vi "unregisterObserverEvent.vi"(8 "error in":errorcluster, 9 "EventReg":refnum<event-registration>, 11 "ObserverClass in":refnum<class "ObserverClass.lvclass">) -> (0 "error out":errorcluster, 3 "ObserverClass out":refnum<class "ObserverClass.lvclass">)   [LabVIEW 2025, in "ObserverClass.lvlib" / "ObserverClass.lvclass"]
doc: "Unregister Observer Event for each Observable"
uses:
  ObserverClass.lvclass
  Controls/observerControl.ctl
  ObserverClass.lvclass/ObserverClass.ctl
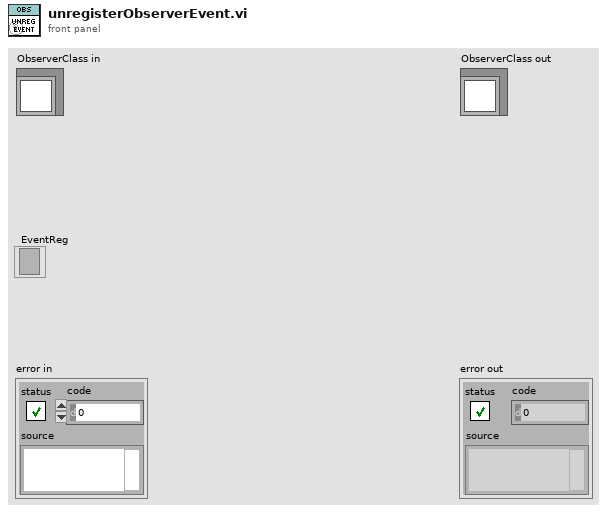
[diagram p1: front panel]
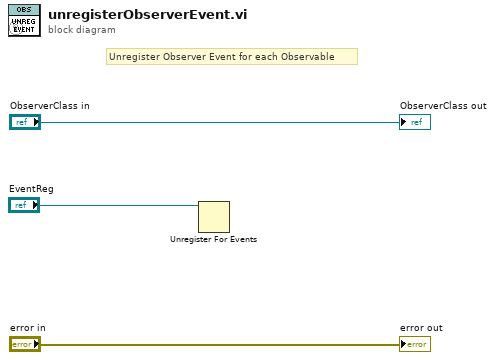
[diagram p0: block diagram]
diagram:
  # "Unregister Observer Event for each Observable"
  n1 = Unregister For Events(event registration refnum="EventReg") -> ()  [unwired: 1 in, 1 out]
  "error out" <- "error in"
  "ObserverClass out" <- "ObserverClass in"
